vi "Forward with Scale.vi"(10 "O Observed Sequence":i32[](array[numeric]), 11 "HMM Cluster":T1) -> (1 "Scale factor":dbl[](array[numeric]), 2 "Scaled Alpha":dbl[][](array[numeric]), 3 "Log10(Prob)":dbl, 5 "Probability":dbl)   [LabVIEW 2014, in "HMM.lvlib"]
doc: "Normalize the partial probability for the forward algorithm."
uses:
  HMM.lvlib
  Control/HMM Cluster.ctl
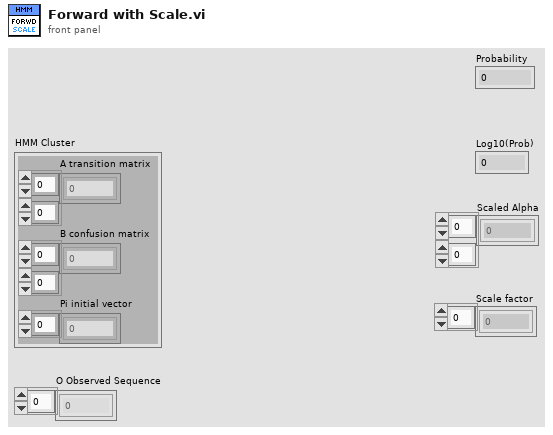
[diagram p1: front panel]
types:
  T1 = typedef "HMM.lvlib/HMM Cluster.ctl" = cluster{"A transition matrix":dbl[][], "B confusion matrix":dbl[][], "Pi initial vector":dbl[]}
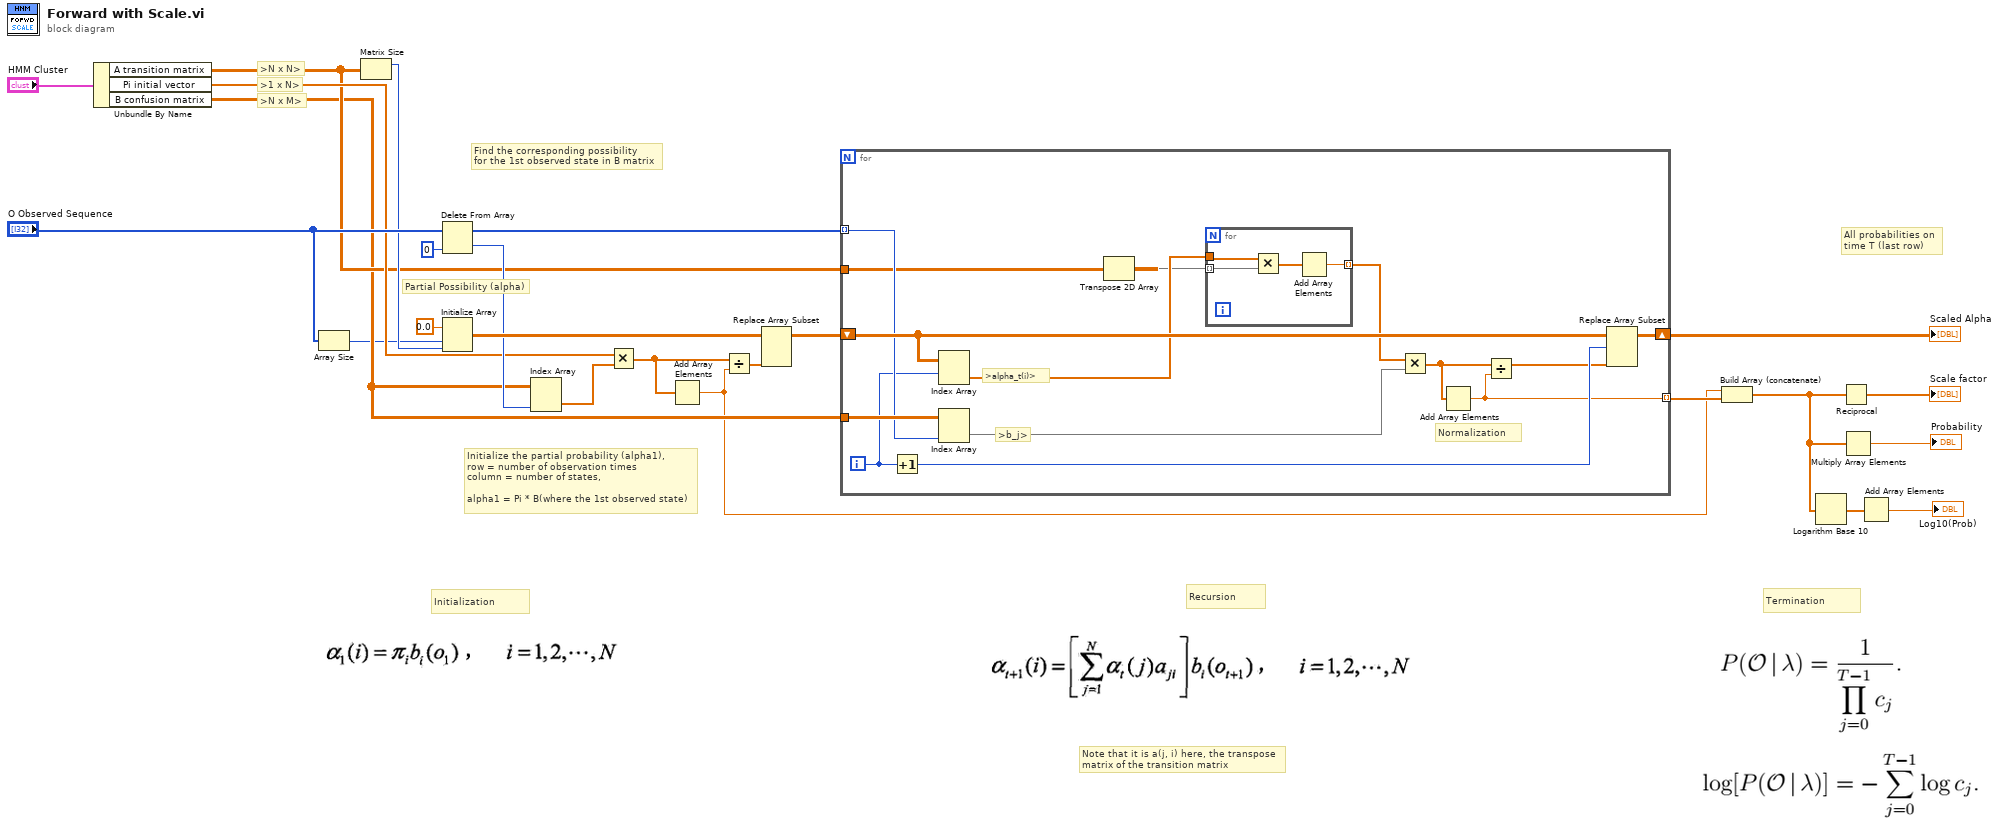
[diagram p0: block diagram]
diagram:
  # "All probabilities on\ntime T (last row)"
  # "Note that it is a(j, i) here, the transpose \nmatrix of the transition matrix"
  # "Termination"
  # "Recursion"
  # "Initialization"
  # ">N x M>"
  # ">1 x N>"
  # ">N x N>"
  # "Partial Possibility (alpha)"
  # "Find the corresponding possibility\nfor the 1st observed state in B matrix"
  # "Initialize the partial probability (alpha1),\nrow = number of observation times\ncolumn = number of states,\n\nalpha1 = Pi * B(where the 1st observed state)"
  n1 = Unbundle By Name("HMM Cluster") -> ("A transition matrix"=w13:dbl[][], "Pi initial vector"=w15:dbl[], "B confusion matrix"=w12:dbl[][])
  n2 = Array Size(array="O Observed Sequence") -> (size(s)=w11:i32)
  n3 = Matrix Size(0:w13) -> (1:w14:i32)  [unwired: 1 out]
  n4 = Delete From Array(array="O Observed Sequence", index=0) -> (deleted portion=w16:i32, array with subset deleted=w18:i32[])  [unwired: 1 in]
  n5 = Initialize Array(0.0 ("element"), w11, w14) -> (w22:dbl[][])
  n6 = Index Array(array=w12, index (col)=w16) -> (element=w19:dbl[])  [unwired: 1 in]
  n7 = Multiply(x=w15, y=w19) -> (x*y=w9:dbl[])
  n8 = Add Array Elements(numeric array=w9) -> (sum=w6:dbl)
  n9 = Divide(x=w9, y=w6) -> (x/y=w8:dbl[])
  n10 = Replace Array Subset(array=w22, new element=w8) -> (w21:dbl[][])  [unwired: 2 in]
  n11 = for {
    tunnel: w18 -> [w34] mode=indexing
    shift-right: [w38] -> w10
    shift-left: w21 -> [w37]
    tunnel: w13 -> [w30]
    tunnel: w12 -> [w35]
    tunnel: [w25] -> w7 mode=indexing
    i -> [w32]
    # "Normalization"
    # ">alpha_t(i)>"
    # ">b_j>"
    n12 = Increment(x=w32) -> (x+1=w36:i32)
    n13 = Index Array(array=w37, index (row)=w32) -> (element=w31:dbl[])  [unwired: 1 in]
    n14 = Index Array(array=w35, index (col)=w34) -> (element=w33:dbl[])  [unwired: 1 in]
    n15 = Transpose 2D Array(2D array=w30) -> (transposed array=w29:dbl[][])
    n16 = for {
      tunnel: w29 -> [w41] mode=indexing
      tunnel: w31 -> [w42]
      tunnel: [w39] -> w28 mode=indexing
      n17 = Multiply(x=w42, y=w41) -> (x*y=w40:dbl[])
      n18 = Add Array Elements(numeric array=w40) -> (sum=w39:dbl)
    }
    n19 = Multiply(x=w28, y=w33) -> (x*y=w27:dbl[])
    n20 = Add Array Elements(numeric array=w27) -> (sum=w25:dbl)
    n21 = Divide(x=w27, y=w25) -> (x/y=w26:dbl[])
    n22 = Replace Array Subset(array=w37, new element=w26, index (row)=w36) -> (w38:dbl[][])  [unwired: 1 in]
  }
  "Scaled Alpha" <- w10
  n23 = Build Array (concatenate)(w6, w7) -> (w3:dbl[])
  n24 = Logarithm Base 10(1:w3) -> (0:w2:dbl[])
  n25 = Reciprocal(x=w3) -> (1/x=→"Scale factor":dbl[])
  n26 = Multiply Array Elements(1:w3) -> (0:→"Probability":dbl)
  n27 = Add Array Elements(numeric array=w2) -> (sum=→"Log10(Prob)":dbl)
